vi "Test1.vi"() -> ()   [LabVIEW 2014]
panel:
  out "波形图表":dbl(graph)
  in  "停止":bool
  in  "手动":bool
  out "液位超限":bool
  in  "设定高度(m)":dbl(slide) scale=0.0..10.0
  in  "调节步长":dbl(knob) scale=0.0..10.0
  out "温度(℃)":dbl(slide) scale=0.0..100.0
  out "压力(MPa)":cluster{dbl, dbl}(knob) scale=0.0..5.0 scale format="%#.2g"
  out "实际液位(m)":dbl(slide) scale=0.0..10.0 scale format="%#.2g"
  # "储蓄罐状态监测"
  # "进口压力"
  # "出口压力"
  # "自动"
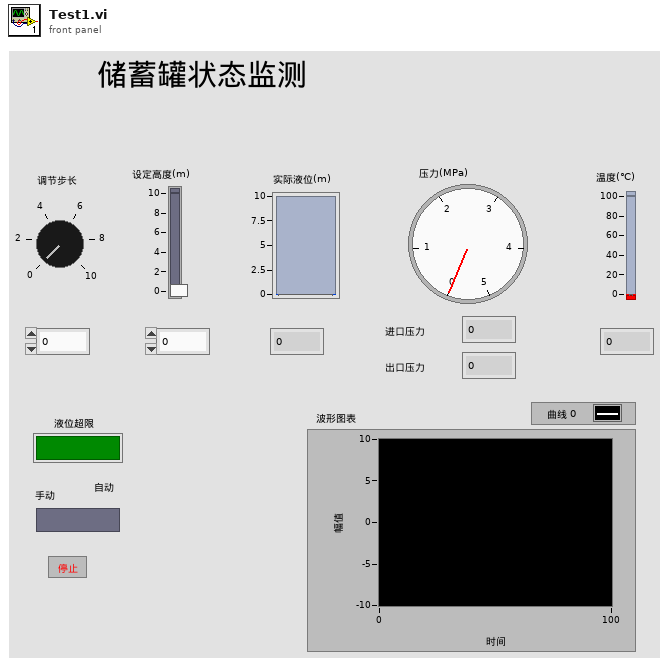
[diagram p1: front panel]
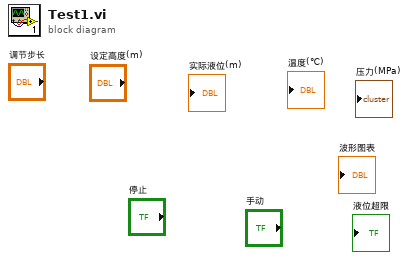
[diagram p0: block diagram]
diagram:
